vi "Calcul ZCR.vi"(11 "ZCR Signal Input":waveform(dbl)[](graph)=[{"t0"=timestamp(3810127384.725 s since 1904-01-01), "dt"=0.0002, "Y"=array[5000 elements]}, {"t0"=timestamp(3810127384.725 s since 1904-01-01), "dt"=0.0002, "Y"=array[5000 elements]}] caption="ZCR signal imput") -> (1 "ZCR Valid":bool, 2 "Controle Decalage":T1 {"Décallage sinus Off" format="%.6f"; "Décallage sinus On" format="%.6f"}, 3 "Reglage decalage":T2={"Delta relais On (Secondes)"=0.009854545454545454, "Delta relais  Off(Secondes)"=0.008963636363636365})   [LabVIEW 2020, in "Library Commun.lvlib" / "Nodon_ZCR.lvclass"]
uses:
  Nodon_ZCR.lvclass
  <vilib>/Analysis/baseanly.llb/Mean (DBL).vi
  <vilib>/measure/mamon.llb/Waveform Peak Detection for 1 Chan.vi
  <vilib>/Analysis/NI_AALBase.lvlib
  <vilib>/measure/NI_MAPro.lvlib
panel:
  # "107,2m"
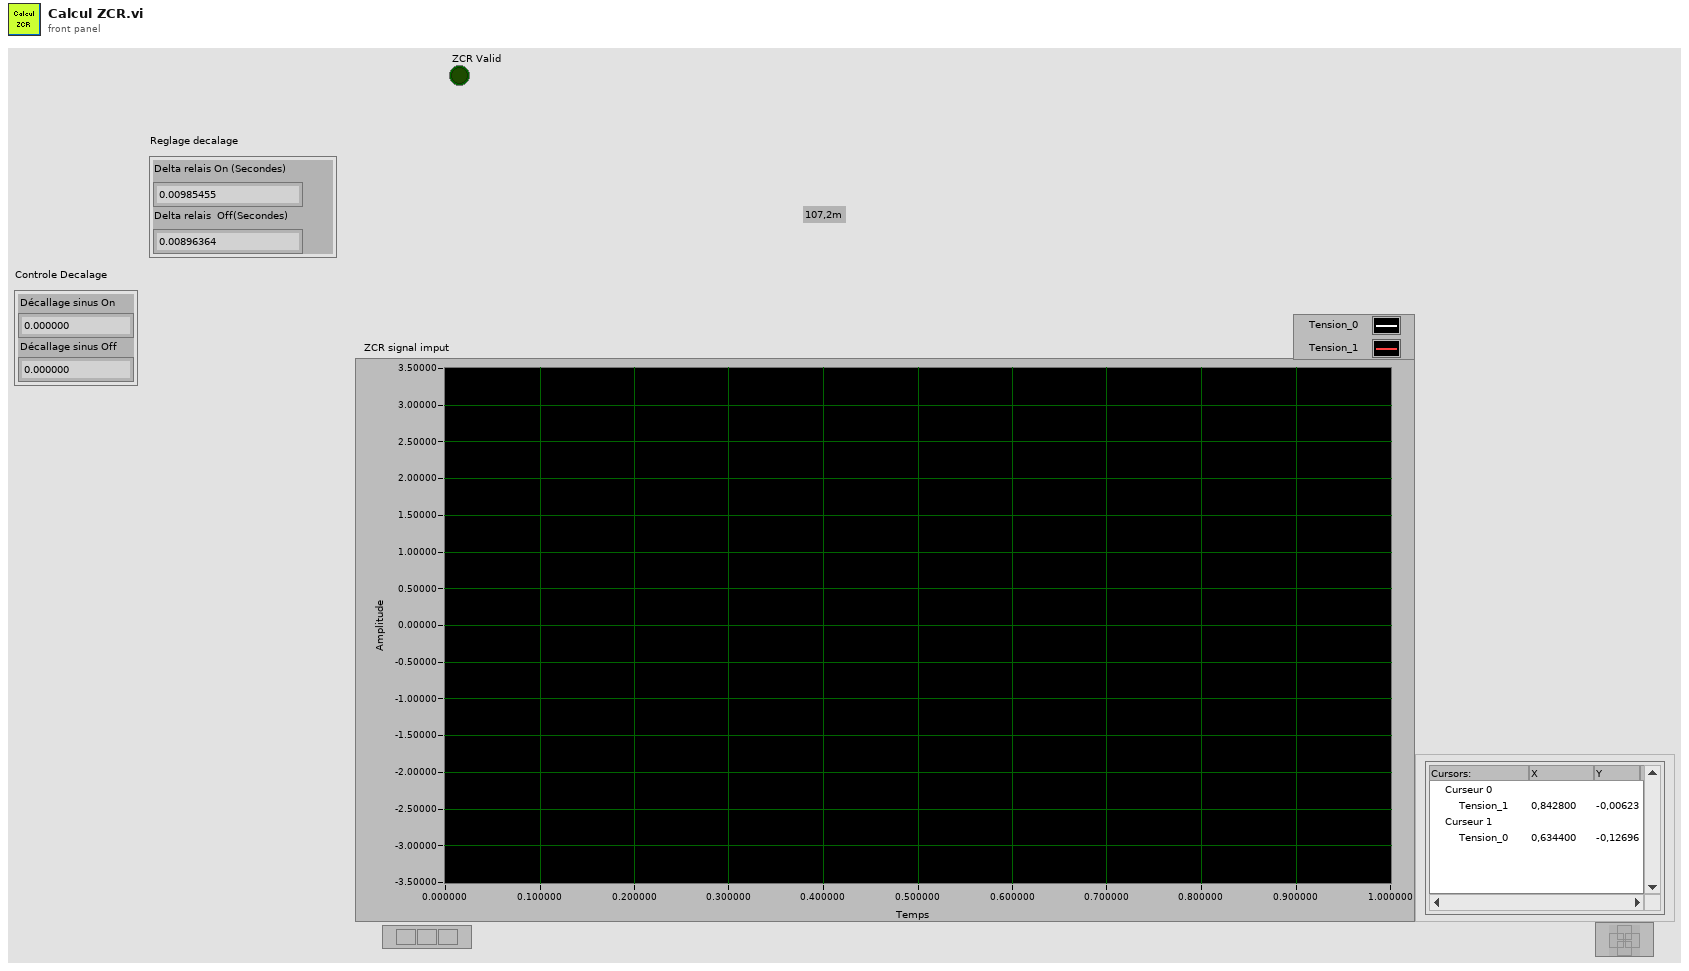
[diagram p1: front panel]
types:
  T1 = cluster{"Décallage sinus On":dbl, "Décallage sinus Off":dbl}
  T2 = cluster{"Delta relais On (Secondes)":dbl, "Delta relais  Off(Secondes)":dbl}
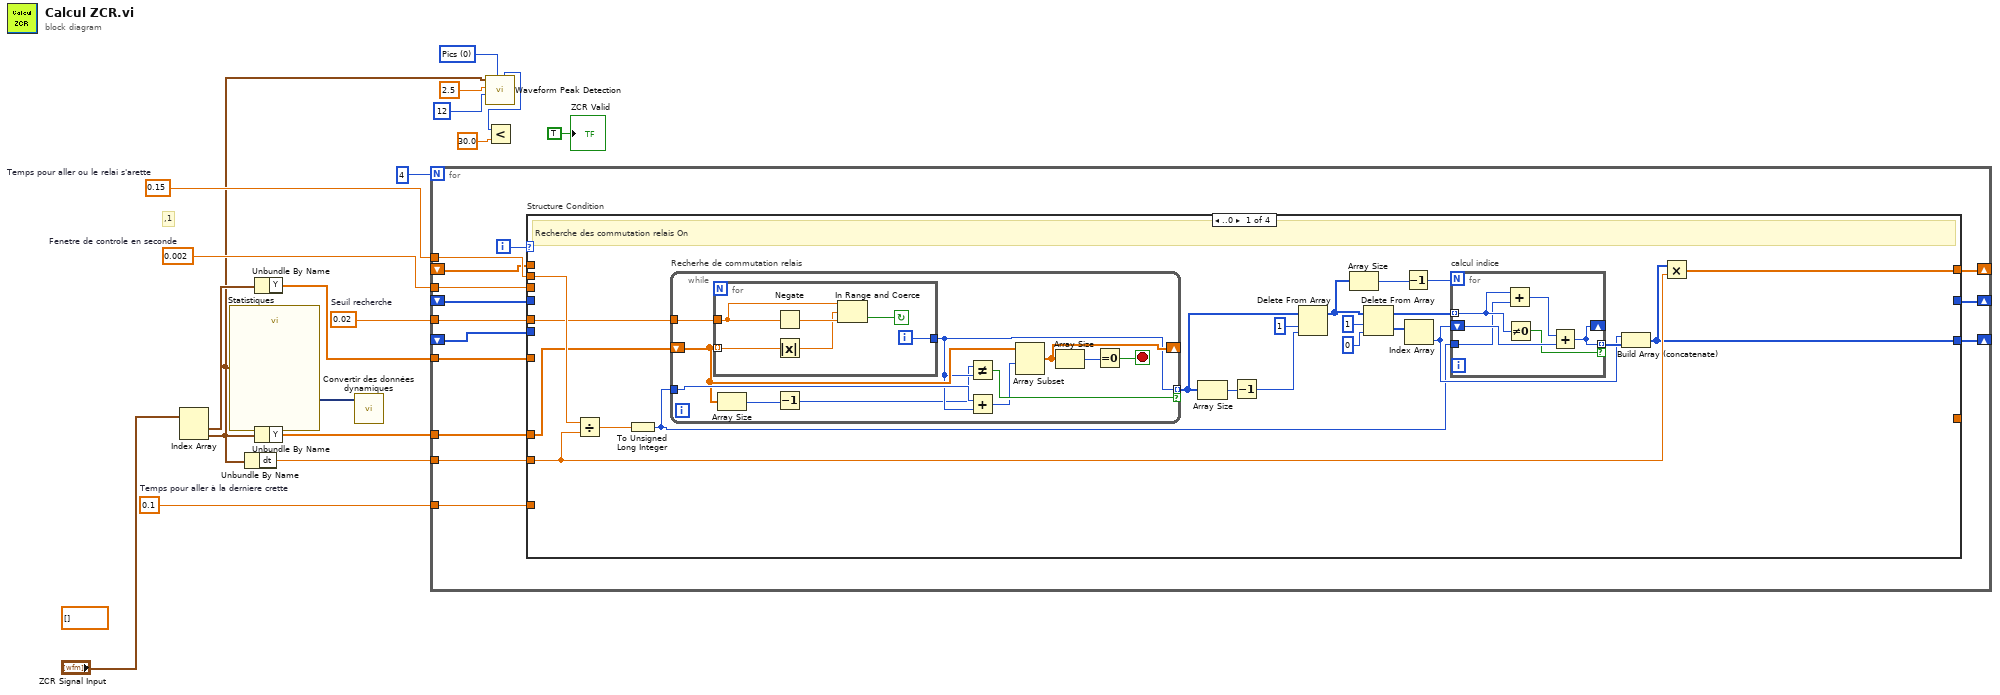
[diagram p0: block diagram]
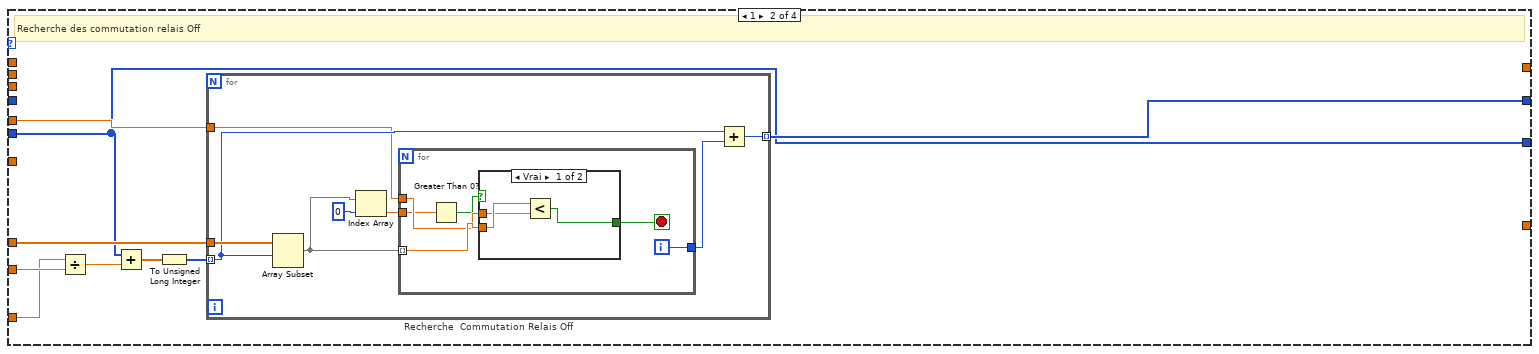
[diagram p2: hidden frame]
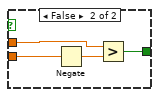
[diagram p3: hidden frame]
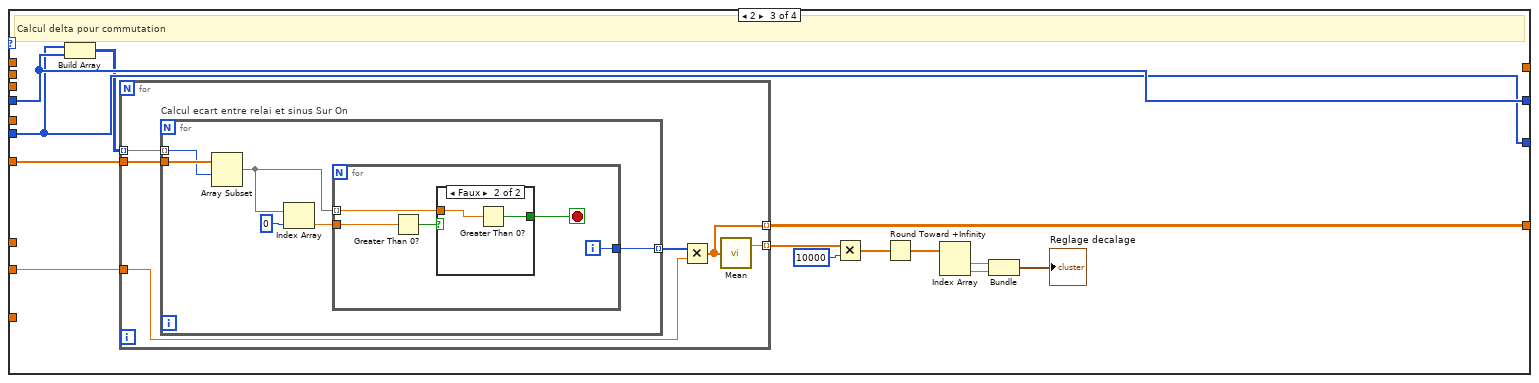
[diagram p4: hidden frame]
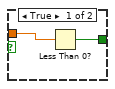
[diagram p5: hidden frame]
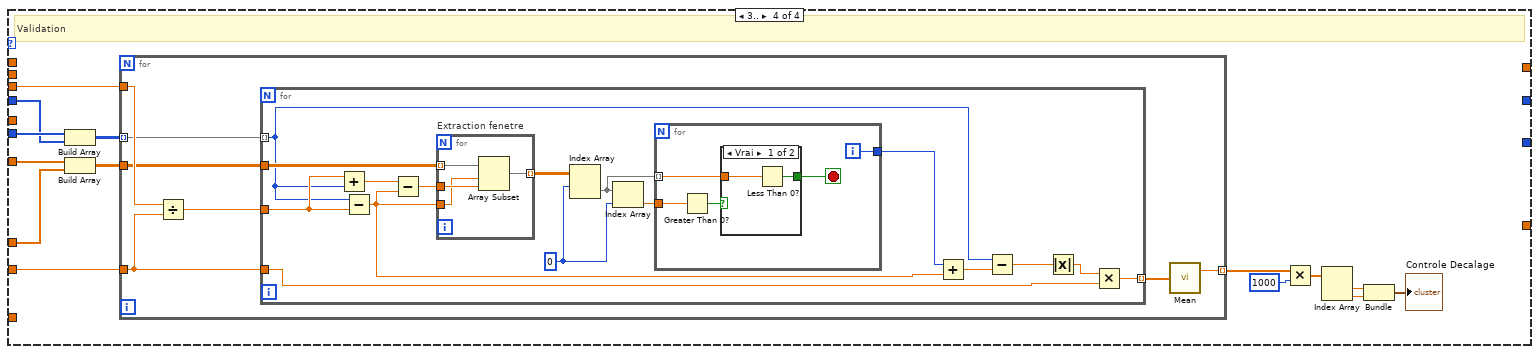
[diagram p6: hidden frame]
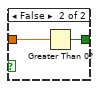
[diagram p7: hidden frame]
diagram:
  w4 = u16 0 items=["Pics", "Vallées"] ("peaks/valleys")
  (unwired) dbl[] [] ("élément")
  w13 = 0.002  # Fenetre de controle en seconde
  w15 = 0.02  # Seuil recherche
  w17 = 0.1  # Temps pour aller à la derniere crette
  w18 = 0.15  # Temps pour aller ou le relai s'arette
  # ",1"
  n1 = Index Array(array="ZCR Signal Input") -> (element #1=w11:waveform(dbl), element #2=w2:waveform(dbl))  [unwired: 2 in]
  n2 = call "Statistiques"("Signals"=w2) -> ("Kurtosis"=w9:dynamicdata)  [unwired: 23 in, 3 out]
  n3 = Unbundle By Name(w2) -> ("dt"=w16:dbl)
  n4 = Unbundle By Name(w11) -> ("Y"=w12:dbl[])
  n5 = Unbundle By Name(w2) -> ("Y"=w8:dbl[])
  n6 = call "Convertir des données dynamiques"("Dynamic Data Type"=w9) -> ()  [unwired: 3 in, 1 out]
  n7 = for {
    N: 4 -> [_]
    tunnel: w18 -> [w32]
    tunnel: w8 -> [w31]
    tunnel: w17 -> [w30]
    tunnel: w16 -> [w29]
    tunnel: w12 -> [w28]
    tunnel: w15 -> [w27]
    shift-right: [w26] -> _
    shift-left: _ -> [w23]
    shift-right: [w25] -> _
    shift-left: _ -> [w24]
    shift-right: [w21] -> _
    shift-left: _ -> [w20]
    tunnel: w13 -> [w19]
    i -> [w22]
    n8 = case "Structure Condition" shown="..0" w22 {
      tunnel: w32 -> [w53 _ _ _]
      tunnel: w31 -> [w42 w82 _ w148]
      tunnel: w30 -> [_ w80 _ _]
      tunnel: w29 -> [w44 w84 w119 w153]
      tunnel: w28 -> [_ _ w118 w149]
      tunnel: w27 -> [w43 w83 _ _]
      tunnel: [w45 _ _ _] -> w26
      tunnel: [w35 w79 w116 _] -> w25
      tunnel: w24 -> [_ w79 w116 w152]
      tunnel: w23 -> [_ _ _ _]
      tunnel: [_ w81 w117 _] -> w21
      tunnel: w20 -> [_ _ w117 w151]
      tunnel: w19 -> [_ _ _ w154]
      tunnel: [_ _ w110 _] -> _
      frame ..0 {
        # "Recherche des commutation relais On"
        n9 = Divide(x=w53, y=w44) -> (x/y=w49:dbl)
        n10 = To Unsigned Long Integer(number=w49) -> (unsigned 32bit integer=w46:u32)
        n11 = while "Recherhe de commutation relais" {
          tunnel: [w65] -> w34 mode=indexing if=w64
          shift-right: [w70] -> _
          shift-left: w42 -> [w67]
          tunnel: w46 -> [w68]
          tunnel: w43 -> [w60]
          stop <- w69 stop-if-true
          n12 = for {
            tunnel: w67 -> [w73] mode=indexing
            tunnel: [w76] -> w65
            tunnel: w60 -> [w75]
            i -> [w76]
            stop <- w72 continue-if-true
            n13 = Negate(x=w75) -> (-x=w74:dbl)
            n14 = Absolute Value(x=w73) -> (abs(x)=w71:dbl)
            n15 = In Range and Coerce(upper limit=w75, x=w71, lower limit=w74) -> (In Range?=w72:bool)  [unwired: 1 out]
          }
          n16 = Array Size(array=w67) -> (size(s)=w66:i32)
          n17 = Decrement(x=w66) -> (x-1=w63:i32)
          n18 = Not Equal?(x=w63, y=w65) -> (x != y?=w64:bool)
          n19 = Add(x=w68, y=w65) -> (x+y=w62:u32)
          n20 = Array Subset(array=w67, index=w62) -> (w70:dbl[])  [unwired: 1 in]
          n21 = Array Size(array=w70) -> (size(s)=w61:i32)
          n22 = Equal To 0?(x=w61) -> (x = 0?=w69:bool)
        }
        n23 = Array Size(array=w34) -> (size(s)=w37:i32)
        n24 = Decrement(x=w37) -> (x-1=w36:i32)
        n25 = Delete From Array(array=w34, length=1 ("longueur"), index=w36) -> (array with subset deleted=w33:i32[])  [unwired: 1 out]
        n26 = Array Size(array=w33) -> (size(s)=w40:i32)
        n27 = Delete From Array(array=w33, length=1 ("longueur"), index=0 ("indice")) -> (deleted portion=w41:i32[], array with subset deleted=w52:i32[])
        n28 = Decrement(x=w40) -> (x-1=w39:i32)
        n29 = Index Array(array=w41) -> (element=w47:i32)  [unwired: 1 in]
        n30 = for "calcul indice" {
          N: w39 -> [_]
          tunnel: w52 -> [w56] mode=indexing
          shift-right: [w57] -> _
          shift-left: w47 -> [w58]
          tunnel: w46 -> [w54]
          tunnel: [w57] -> w48 mode=indexing if=w55
          n31 = Add(x=w56, y=w54) -> (x+y=w59:u32)
          n32 = Not Equal To 0?(x=w56) -> (x != 0?=w55:bool)
          n33 = Add(x=w59, y=w58) -> (x+y=w57:u32)
        }
        n34 = Build Array (concatenate)(w47, w48) -> (w35:u32[])
        n35 = Multiply(x=w35, y=w44) -> (x*y=w45:dbl[])
      }
      frame 1 {
        # "Recherche des commutation relais Off"
        n36 = Divide(x=w80, y=w84) -> (x/y=w78:dbl)
        n37 = Add(x=w79, y=w78) -> (x+y=w77:dbl[])
        n38 = To Unsigned Long Integer(number=w77) -> (unsigned 32bit integer=w85:u32[])
        n39 = for "Recherche  Commutation Relais Off" {
          tunnel: [w90] -> w81 mode=indexing
          tunnel: w85 -> [w91] mode=indexing
          tunnel: w82 -> [w92]
          tunnel: w83 -> [w89]
          n40 = Array Subset(array=w92, index=w91) -> (w87:dbl[])  [unwired: 1 in]
          n41 = Index Array(array=w87, index=0 ("indice")) -> (element=w86:dbl)
          n42 = for {
            tunnel: w87 -> [w99] mode=indexing
            tunnel: [w97] -> w93
            tunnel: w89 -> [w96]
            tunnel: w86 -> [w95]
            i -> [w97]
            stop <- w98 stop-if-true
            n43 = Greater Than 0?(x=w95) -> (x > 0?=w94:bool)
            n44 = case shown="Vrai" w94 {
              tunnel: w99 -> [w102 w106]
              tunnel: [w101 w105] -> w98
              tunnel: w96 -> [w100 w104]
              frame True {
                n45 = Less?(x=w102, y=w100) -> (x < y?=w101:bool)
              }
              frame False {
                n46 = Negate(x=w106) -> (-x=w103:dbl)
                n47 = Greater?(x=w104, y=w103) -> (0:w105:bool)
              }
            }
          }
          n48 = Add(x=w91, y=w93) -> (x+y=w90:u32)
        }
      }
      frame 2 {
        # "Calcul delta pour commutation"
        n49 = Build Array(w116, w117) -> (w115:u32[][])
        n50 = for {
          tunnel: [w125] -> w114 mode=indexing
          tunnel: w119 -> [w123]
          tunnel: w118 -> [w122]
          tunnel: w115 -> [w121] mode=indexing
          tunnel: [w120] -> w110 mode=indexing
          n51 = for "Calcul ecart entre relai et sinus Sur On" {
            tunnel: w121 -> [w130] mode=indexing
            tunnel: w122 -> [w131]
            tunnel: [w129] -> w124 mode=indexing
            n52 = Array Subset(array=w131, index=w130) -> (w128:dbl[])  [unwired: 1 in]
            n53 = Index Array(array=w128, index=0 ("indice")) -> (element=w126:dbl)
            n54 = for {
              tunnel: w128 -> [w136] mode=indexing
              tunnel: [w134] -> w129
              tunnel: w126 -> [w133]
              i -> [w134]
              stop <- w135 stop-if-true
              n55 = Greater Than 0?(x=w133) -> (x > 0?=w132:bool)
              n56 = case shown="Faux" w132 {
                tunnel: w136 -> [w138 w140]
                tunnel: [w137 w139] -> w135
                frame True {
                  n57 = Less Than 0?(x=w138) -> (x < 0?=w137:bool)
                }
                frame False {
                  n58 = Greater Than 0?(x=w140) -> (x > 0?=w139:bool)
                }
              }
            }
          }
          n59 = Multiply(x=w124, y=w123) -> (x*y=w120:dbl[])
          n60 = call-poly <vilib>:"Mean.vi"("X"=w120) -> ("mean"=w125:dbl)  [unwired: 1 out]
        }
        n61 = Multiply(x=w114, y=10000) -> (x*y=w109:dbl[])
        n62 = Round Toward +Infinity(x=w109) -> (ceil(x): smallest int >= x=w107:dbl[])
        n63 = Index Array(array=w107) -> (element #1=w113:dbl, element #2=w112:dbl)  [unwired: 2 in]
        n64 = Bundle(w113, w112) -> (→"Reglage decalage":cluster{dbl, dbl})  [unwired: 1 in]
      }
      frame 3.. {
        # "Validation"
        n65 = Build Array(w152, w151) -> (w150:u32[][])
        n66 = Build Array(w149, w148) -> (w144:dbl[][])
        n67 = for {
          tunnel: w154 -> [w161]
          tunnel: w150 -> [w160] mode=indexing
          tunnel: w153 -> [w157]
          tunnel: w144 -> [w158]
          tunnel: [w156] -> w142 mode=indexing
          n68 = Divide(x=w161, y=w157) -> (x/y=w159:dbl)
          n69 = for {
            tunnel: w160 -> [w163] mode=indexing
            tunnel: w159 -> [w166]
            tunnel: w158 -> [w177]
            tunnel: w157 -> [w176]
            tunnel: [w175] -> w155 mode=indexing
            w169 = 0 ("indice")
            n70 = Add(x=w166, y=w163) -> (x+y=w167:dbl)
            n71 = Subtract(x=w163, y=w166) -> (x-y=w164:dbl)
            n72 = Subtract(x=w167, y=w164) -> (x-y=w165:dbl)
            n73 = for "Extraction fenetre" {
              tunnel: w177 -> [w190] mode=indexing
              tunnel: [w189] -> w171 mode=indexing
              tunnel: w165 -> [w188]
              tunnel: w164 -> [w187]
              n74 = Array Subset(array=w190, index=w187, length=w188) -> (w189:dbl[])
            }
            n75 = Index Array(array=w171, index (row)=w169) -> (element=w170:dbl[])  [unwired: 1 in]
            n76 = Index Array(array=w170, index=w169) -> (element=w173:dbl)
            n77 = for {
              tunnel: w170 -> [w182] mode=indexing
              tunnel: w173 -> [w179]
              tunnel: [w178] -> w172
              i -> [w178]
              stop <- w181 stop-if-true
              n78 = Greater Than 0?(x=w179) -> (x > 0?=w180:bool)
              n79 = case shown="Vrai" w180 {
                tunnel: w182 -> [w184 w186]
                tunnel: [w183 w185] -> w181
                frame True {
                  n80 = Less Than 0?(x=w184) -> (x < 0?=w183:bool)
                }
                frame False {
                  n81 = Greater Than 0?(x=w186) -> (x > 0?=w185:bool)
                }
              }
            }
            n82 = Add(x=w172, y=w164) -> (x+y=w168:dbl)
            n83 = Subtract(x=w163, y=w168) -> (x-y=w162:dbl)
            n84 = Absolute Value(x=w162) -> (abs(x)=w174:dbl)
            n85 = Multiply(x=w174, y=w176) -> (x*y=w175:dbl)
          }
          n86 = call-poly <vilib>:"Mean.vi"("X"=w155) -> ("mean"=w156:dbl)  [unwired: 1 out]
        }
        n87 = Multiply(x=w142, y=1000) -> (x*y=w141:dbl[])
        n88 = Index Array(array=w141) -> (element #1=w147:dbl, element #2=w146:dbl)  [unwired: 2 in]
        n89 = Bundle(w147, w146) -> (→"Controle Decalage":cluster{dbl, dbl})  [unwired: 1 in]
      }
    }
  }
  n90 = call-poly <vilib>:"Waveform Peak Detection.vi"("peaks/valleys"=w4, "width"=12, "threshold"=2.5, "Signal In"=w2) -> ("# found"=w3:i32)  [unwired: 3 in, 4 out]
  n91 = Less?(x=w3, y=30.0) -> ()  [unwired: 1 out]
  "ZCR Valid" <- TRUE ("ZCR Valid")
